vi "Read Packet.vi"(8 "error in (no error)":errorcluster, 11 "MQTT_Base in":refnum<class "MQTT_Base.lvclass">) -> (0 "error out":errorcluster, 1 "SessionMailbox":refnum<queue>, 2 "Packet":refnum<class "ControlPacket.lvclass">, 3 "MQTT_Base out":refnum<class "MQTT_Base.lvclass">)   [LabVIEW 2013, in "MQTT Base.lvlib" / "MQTT_Base.lvclass"]
uses:
  MQTT_Base.lvclass
  <vilib>/LabVIEW Open Source Project/MQTT Control Packets/Control Packets/ControlPacket/ControlPacket.lvclass
  Response -- cluster.ctl
  MQTT_Base.lvclass/MQTT_Base.ctl
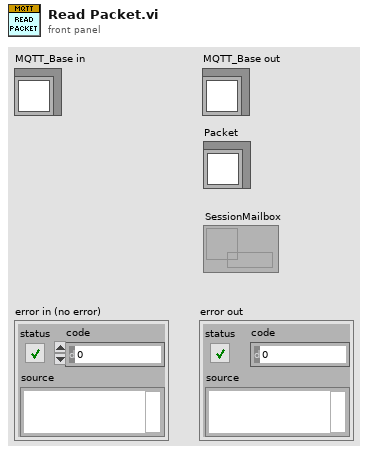
[diagram p1: front panel]
types:
  T1 = typedef "MQTT Server.lvlib/MQTT_Base.lvclass/Request -- cluster.ctl" = cluster{"Packet":refnum<class "ControlPacket.lvclass">, "SessionMailbox":refnum<queue>}
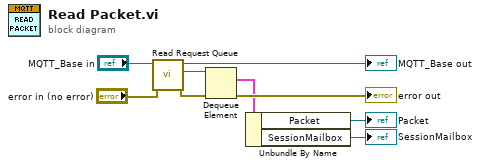
[diagram p0: block diagram]
diagram:
  n1 = call "Read Request Queue.vi"("error in (no error)"="error in (no error)", "MQTT_Base in"="MQTT_Base in") -> ("error out"=w2:errorcluster, "Request"=w1:refnum<queue>, "MQTT_Base out"=→"MQTT_Base out":refnum<class "MQTT_Base.lvclass">)  [unwired: 7 in]
  n2 = Dequeue Element(queue=w1, error in (no error)=w2) -> (element=w5:T1, error out=→"error out":errorcluster)  [unwired: 1 in, 2 out]
  n3 = Unbundle By Name(w5) -> ("Packet"=→"Packet":refnum<class "ControlPacket.lvclass">, "SessionMailbox"=→"SessionMailbox":refnum<queue>)
